vi "OAT Resample Waveform (Single Channel).vi"(5 "reset? (True)":bool=TRUE, 6 "max order (auto)":i32, 7 "A stop (72 dB)":dbl=72.0, 8 "error in (no error)":errorcluster, 9 "pulse/revolution (1)":i32=1, 10 "speed profile":T4 {"speed [RPM]" format="%.2f"; "time [s]" format="%.2f"}, 11 "scaled signal [EU]":waveform(dbl)={"t0"=timestamp(0 s since 1904-01-01), "dt"=0.0, "Y"=[]}) -> (0 "error out":errorcluster, 1 "interpolated pulse positions":dbl[](array[numeric]) format="%.2f", 2 "channel info":T1={"sensor sensitivity"=1000.0, "engineering units"=1, "dB reference"=1.0, "custom label"="EU", "weighting filter"=0, "pregain"=0.0} {"pregain" format="%.2f"; "weighting filter" items=["Linear", "A-weighting", "B-weighting", "C-weighting", "ITU-R 468-4", "Dolby", "CCITT", "C-message", "Wb", "Wc", "Wd", "We", "Wf", "Wh", "Wj", "Wk", "Wm", "AES17 20 kHz lowpass", "AES17 40 kHz lowpass", "AES17 20 kHz highpass", "AES17 40 kHz highpass"]; "dB reference" format="%^.1e"; "engineering units" items=["custom..."=0, "V"=1, "A"=21, "C"=30, "pC"=31, "s"=32, "-"=29, "Pa"=2, "N"=20, "g"=3, "m/s^2"=4, "m/s"=5, "m"=6, "mm/s"=12, "mm"=13, "micron/s"=14, "micron"=15, "in/s^2"=7, "in/s"=8, "in"=9, "mil/s"=10, "mil"=11, "rad/s^2"=16, "rad/s"=17, "rad"=18, "deg/s^2"=26, "deg/s"=27, "deg"=28, "RPM"=22, "cycle/s^2"=23, "Hz"=24, "cycle"=25, "strain"=19]; "sensor sensitivity" format="%#_5f"}, 3 "resampled signal":cluster{"r0":dbl, "dr":dbl, "Y":dbl[]}={"r0"=0.0, "dr"=1.0, "Y"=[]} {"r0" format="%.2p"; "dr" format="%.2p"; "Y" format="%.2f"})   [LabVIEW 2017]
doc: "Resample the even time sampled <B>scaled signal [EU]</B> to even angle sampled signal."
uses:
  <vilib>/addons/Sound and Vibration/Order Analysis/Tach Process/SubVIs/speed profile.ctl
  <vilib>/addons/_NISVFA/_Shared subVIs/Controls/svc_Channel Info.ctl
  <vilib>/addons/_NISVFA/_Shared subVIs/Controls/svc_Engineering Units Text Ring.ctl
  <vilib>/addons/_NISVFA/_Shared subVIs/Controls/svc_Weighting Filter Text Ring.ctl
  <vilib>/addons/Sound and Vibration/Order Analysis/Adv Resampling/oa_Adjust Resample State Info.vi
  <vilib>/addons/Sound and Vibration/Order Analysis/Misc/OAT Error Information.vi
  <vilib>/addons/Sound and Vibration/Order Analysis/Adv Resampling/OAT Prepare Resample Data.vi
  <vilib>/addons/_NISVFA/_Shared subVIs/Common/svc_Engineering Units to Unit Label.vi
  <vilib>/addons/_NISVFA/_Shared subVIs/Common/svc_Unit Label to Engineering Units.vi
  <vilib>/addons/Sound and Vibration/Order Analysis/Resample Order Tracking/SoundVib_Resampling.lvlib
  <vilib>/addons/Sound and Vibration/Order Analysis/Tach Process/SoundVib_TachProcess.lvlib
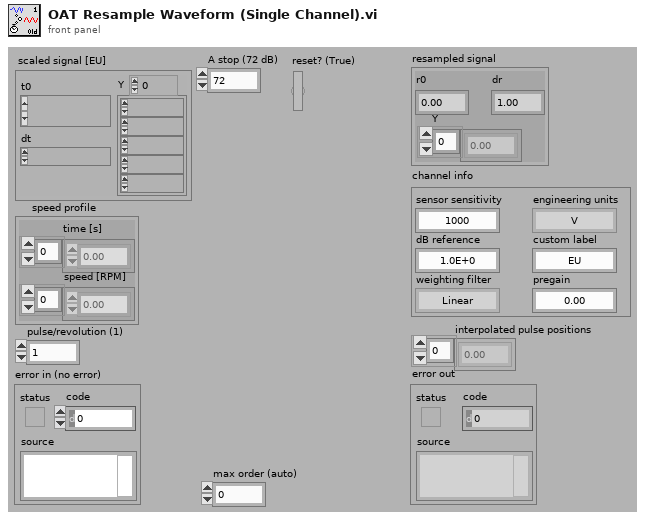
[diagram p1: front panel]
types:
  T1 = typedef "svc_Channel Info.ctl" = cluster{"sensor sensitivity":dbl, "engineering units":T2, "dB reference":dbl, "custom label":string, "weighting filter":T3, "pregain":dbl}
  T2 = typedef "svc_Engineering Units Text Ring.ctl" = u16
  T3 = typedef "svc_Weighting Filter Text Ring.ctl" = u16
  T4 = typedef "SoundVib_TachProcess.lvlib/speed profile.ctl" = cluster{"time [s]":dbl[], "speed [RPM]":dbl[]}
  T5 = typedef "OAT Resample Filter Prototype.ctl" = cluster{"left wing":dbl[], "increment":dbl[], "max dec":i32, "timing jitter":enum32{"Interpolation", "Rounding"}, "band limiting?":bool}
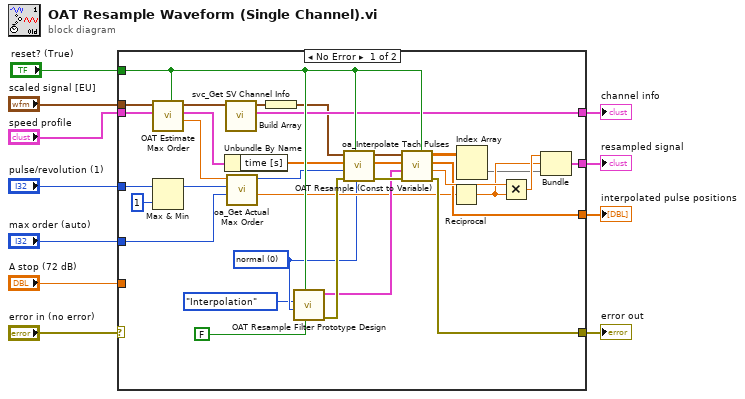
[diagram p0: block diagram]
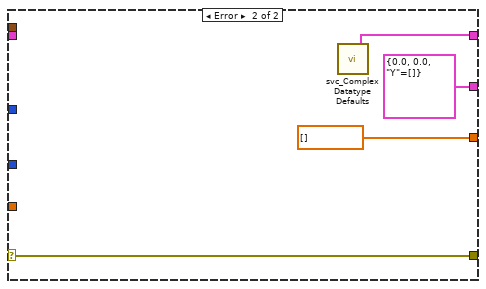
[diagram p2: hidden frame]
diagram:
  n1 = case shown="No Error" "error in (no error)" {
    selector: "error in (no error)" -> [_ w45]
    tunnel: "pulse/revolution (1)" -> [w43 _]
    tunnel: "max order (auto)" -> [w42 _]
    tunnel: [w41 cluster{dbl, dbl, "Y":dbl[]} {0.0, 0.0, "Y"=[]}] -> w9
    tunnel: "scaled signal [EU]" -> [w36 _]
    tunnel: "speed profile" -> [w35 _]
    tunnel: [w32 dbl[] [] ("time stamps")] -> w6
    tunnel: "reset? (True)" -> [w24 _]
    tunnel: [w31 w45] -> w4
    tunnel: "A stop (72 dB)" -> [_ _]
    tunnel: [w18 w44] -> w1
    frame No Error {
      w17 = u16 0 items=["normal", "high"] ("resolution")
      n2 = call <vilib>:"OAT Estimate Max Order.vi"("reset? (True)"=w24, "speed profile in"=w35, "scaled signal [EU] in"=w36) -> ("max suggested order"=w33:dbl, "speed profile out"=w34:T4, "scaled signal [EU] out"=w20:waveform(dbl))  [unwired: 5 in, 1 out]
      n3 = Max & Min(x=w43, y=1) -> (max(x,y)=w22:i32)  [unwired: 1 out]
      n4 = Unbundle By Name(w34) -> ("time [s]"=w15:dbl[])
      n5 = call <vilib>:"svc_Get SV Channel Info.vi"("scaled signal [EU]"=w20) -> ("channel info"=w18:T1, "dup scaled signal [EU]"=w19:waveform(dbl))  [unwired: 5 in, 4 out]
      n6 = call <vilib>:"oa_Get Actual Max Order.vi"("max order (auto)"=w42, "pulse/revolution (1)"=w22, "max suggested order"=w33) -> ("new pulse/revolution"=w21:dbl, "interpolation factor"=w23:i32)  [unwired: 7 in]
      n7 = Build Array(w19) -> (w12:waveform(dbl)[])
      n8 = call <vilib>:"OAT Resample Filter Prototype Design.vi"("alias free"=FALSE ("alias protect in final transition"), "reset? (True)"=w24, "resolution"=w17, "timing jitter"=enum32{"Interpolation", "Rounding"}."Interpolation") -> ("error out"=w30:errorcluster, "filter prototype"=w27:T5)  [unwired: 5 in, 1 out]
      n9 = call <vilib>:"oa_Interpolate Tach Pulses.vi"("resolution"=w17, "reset? (True)"=w24, "error in (no error)"=w30, "interpolation factor"=w23, "pulse positions [s]"=w15, "scaled signals (EU)"=w12) -> ("error out"=w29:errorcluster, "interpolated pulse positions[s]"=w13:dbl[], "dup scaled signals (EU)"=w14:waveform(dbl)[])  [unwired: 2 in, 1 out]
      n10 = call <vilib>:"OAT Resample (Const to Variable).vi"("reset? (True)"=w24, "error in (no error)"=w29, "filter prototype"=w27, "time"=w13, "scaled signals (EU)"=w14) -> ("error out"=w31:errorcluster, "offset"=w38:dbl, "time stamps"=w32:dbl[], "Y"=w25:dbl[][])  [unwired: 3 in]
      n11 = Reciprocal(x=w21) -> (1/x=w37:dbl)
      n12 = Index Array(array=w25) -> (element=w26:dbl[])  [unwired: 2 in]
      n13 = Multiply(x=w38, y=w37) -> (x*y=w39:dbl)
      n14 = Bundle(w39, w37, "Y"=w26) -> (w41:cluster{dbl, dbl, "Y":dbl[]})  [unwired: 1 in]
    }
    frame Error {
      n15 = call <vilib>:"svc_Complex Datatype Defaults.vi"() -> ("channel info"=w44:T1)  [unwired: 11 in, 8 out]
    }
  }
  "resampled signal" <- w9
  "channel info" <- w1
  "interpolated pulse positions" <- w6
  "error out" <- w4
